vi "FXP_LinearControlLaw_singleAxis_uk_and_deltauk.vi"(10 "setpoint":fxp<+/-,32,5>, 11 "ControlParams_distEst":T1={"umax"=3.0, "Ns_obs/cntrl"=0, "du_max"=0.0, "Nbar"=0.0, "Nhyst"=0, "Nsat"=0, "Ndrift+1"=0, "Ki-y"=0.01, "Ns_xff+1"=0, "Ns_yff+1"=0, "Ns_Dx+1"=0, "Ns_Dy+1"=0}) -> (0 "del u_x":fxp<+/-,64,15>, 2 "u_k (un saturated)":fxp<+/-,32,5>)   [LabVIEW 2017]
uses:
  typeDefs/FXPControlParams-ss-xy.ctl
  <vilib>/Platform/TimedLoop/XDataNode/timing_clust.ctl
  <vilib>/Platform/TimedLoop/XDataNode/nitl_modes.ctl
  <vilib>/Platform/TimedLoop/XDataNode/wakeup.ctl
  <vilib>/rvi/Emulation/niFpgaSctlEmulationGetInTimedLoop.vi
  <vilib>/rvi/Emulation/niFpgaEmulationReportErrorSimple.vi
  <vilib>/rvi/Emulation/niFpgaGetClockAttributes.vi
  <vilib>/rvi/Emulation/niFpgaCriticalErrorInLSC.vi
  <vilib>/Platform/TimedLoop/XDataNode/XDataNode.xnode
  <vilib>/rvi/FXPMathLib/FxpAdd/XNode/nifxpmath_Add.xnode
  <vilib>/Platform/TimedLoop/XDataNode/XDNodeRunTimeDep.lvlib
  <vilib>/rvi/FXPMathLib/sim/FxpSim.dll
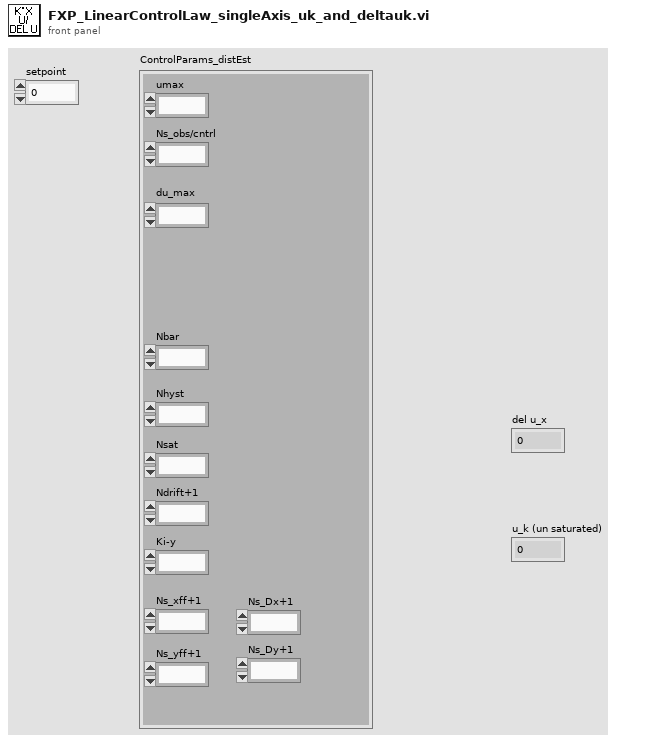
[diagram p1: front panel]
types:
  T1 = typedef "FXPControlParams-ss-xy.ctl" = cluster{"umax":fxp<+/-,18,5>, "Ns_obs/cntrl":u8, "du_max":fxp<+/-,18,5>, "Nbar":fxp<+/-,32,5>, "Nhyst":u8, "Nsat":u8, "Ndrift+1":u8, "Ki-y":sgl, "Ns_xff+1":u8, "Ns_yff+1":u8, "Ns_Dx+1":u8, "Ns_Dy+1":u8}
  T2 = typedef "XDNodeRunTimeDep.lvlib/timing_clust.ctl" = cluster{"Expected End [f-1]":u64, "Actual End [f-1]":u64, "Finished Late? [f-1]":bool, "Expected End [i-1]":u64, "Actual End [i-1]":u64, "Finished Late? [i-1]":bool, "Expected Start [i]":u64, "Actual Start [i]":u64, "Expected Start [f]":u64, "Actual Start [f]":u64, "Source Name":string, "Structure Name":string, "Period":i64, "Deadline":i64, "Offset":i64, "Start":i64, "Priority":i32, "Timeout":i32, "Mode":T3, "Wakeup Reason":T4, "Error":errorcluster, "Source Type":string, "Secondary Source Type":string, "Global End Time":u64, "Global Start Time":u64, "Frame Duration":u64, "Iteration Duration":u64, "Assigned CPU":i32, "I/O Scan Engine Mode":u32}
  T3 = typedef "XDNodeRunTimeDep.lvlib/nitl_modes.ctl" = enum32{"No Change", "Process missed periods, maintain original phase", "Discard missed periods, maintain original phase", "Process missed periods, ignore original phase", "Discard missed periods, ignore original phase"}
  T4 = typedef "XDNodeRunTimeDep.lvlib/wakeup.ctl" = enum32{"Normal", "Aborted", "Asynchronous wakeup", "Timing source error", "Timed loop error", "Timeout"}
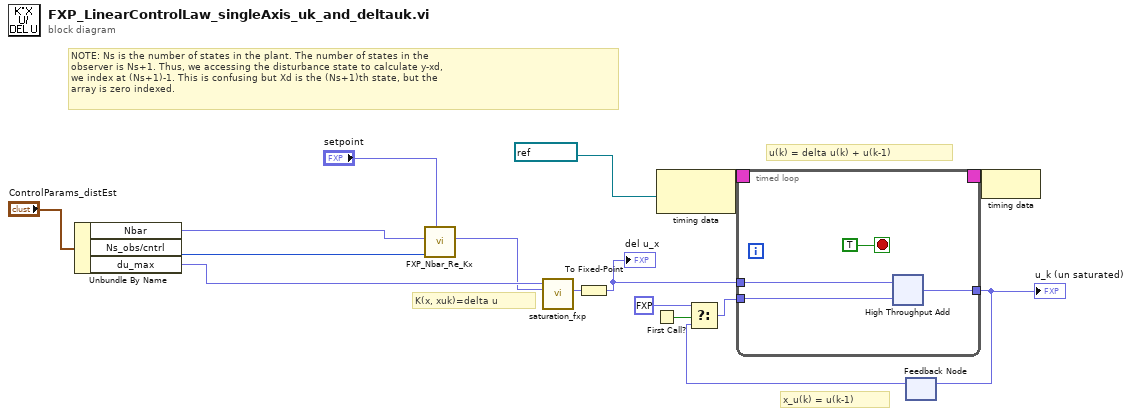
[diagram p0: block diagram]
diagram:
  # "K(x, xuk)=delta u"
  # "u(k) = delta u(k) + u(k-1)"
  # "x_u(k) = u(k-1)"
  # "NOTE: Ns is the number of states in the plant. The number of states in the \nobserver is Ns+1. Thus, we accessing the disturbance state to calculate y-xd, \nwe index at (Ns+1)-1. This is confusing but Xd is the (Ns+1)th state, but the \narray is zero indexed."
  n1 = Unbundle By Name("ControlParams_distEst") -> ("Nbar"=w7:fxp<+/-,32,5>, "Ns_obs/cntrl"=w8:u8, "du_max"=w10:fxp<+/-,18,5>)
  n2 = call "FXP_Nbar_Re_Kx.vi"("ref"="setpoint", "NS"=w8, "Nbar"=w7) -> ("del u_x"=w9:fxp<+/-,32,16>)  [unwired: 8 in]
  n3 = call "saturation_fxp.vi"("uMax"=w10, "signal_in"=w9) -> ("signal_out (saturated)"=w11:fxp<+/-,18,5>)  [unwired: 8 in, 1 out]
  n4 = To Fixed-Point(number=w11) -> (fixed-point=w15:fxp<+/-,32,6>)  [unwired: 1 in]
  "del u_x" <- w15
  n5 = First Call?() -> (First Call?: T/F=w5:bool)
  n6 = node-c288(refnum<k21> "80MHz" ("Source Name")) -> (w14:T2)
  n7 = feedback #1() -> (w4:fxp<+/-,32,5>)  [unwired: 1 in]
  n8 = Select(t=fxp<+/-,32,5> 0.0, s=w5, f=w4) -> (s? t:f=w3:fxp<+/-,32,5>)
  n9 = timed-loop {
    timing: w14 -> [_]
    timing-out: [_] -> w13
    tunnel: [w19] -> w6
    tunnel: w15 -> [w20]
    tunnel: w3 -> [w18]
    stop <- TRUE stop-if-true
    n10 = xnode ("High Throughput Add")("x"=w20, "y"=w18) -> ("x+y"=w19:fxp<+/-,32,5>)
  }
  "u_k (un saturated)" <- w6
  n11 = feedback-in #1(w6) -> ()
  n12 = node-c288(w13) -> ()
